vi "EditorDaemon openFile.vi"(8 "error in (no error)":errorcluster, 9 "dataName":string(combo) caption="Data Name", 10 "filePath":path caption="File Path") -> (0 "error out":errorcluster, 1 "dataName out":string caption="Data Name", 2 "currFilePath":path, 3 "signal out":waveform(sgl), 4 "update":bool)   [LabVIEW 2018]
uses:
  PC/PublicSubVI/Class/FileManager/FM/ctl/_PC_Pub_FM fileReadFuncEnum.ctl
  PC/PublicSubVI/Class/FileManager/TDMSAdv.lvclass
panel:
  out "remark":string caption="Data Remark"
  in  "cancelBtn":bool
  in  "loadBtn":bool
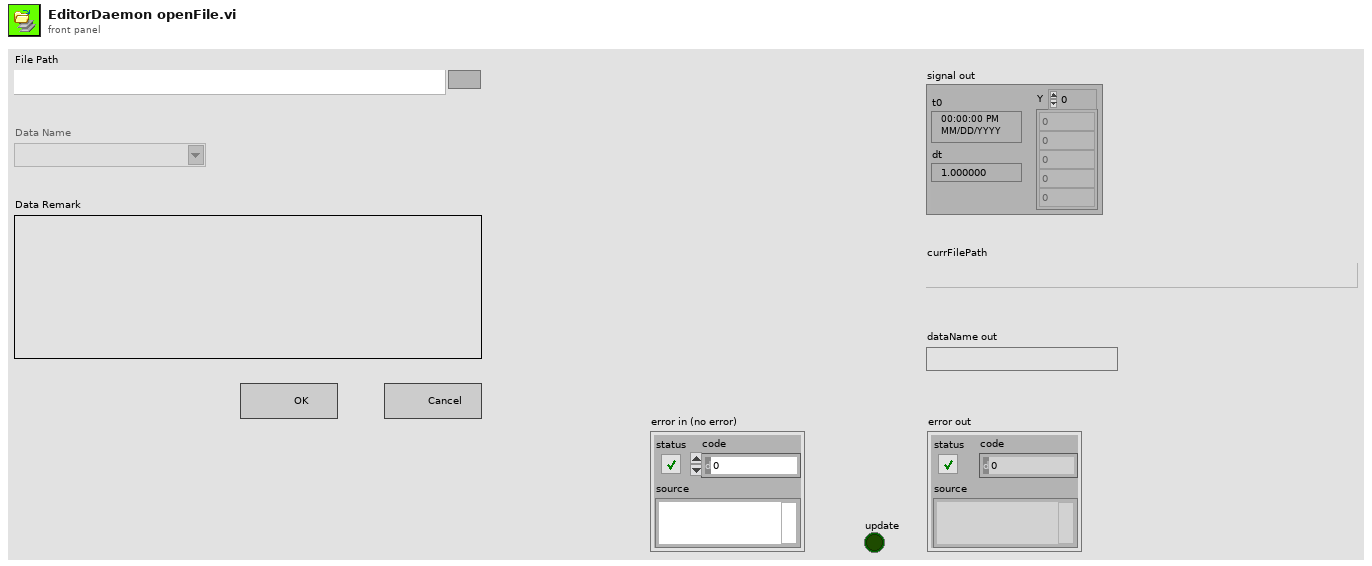
[diagram p1: front panel]
types:
  T1 = enum8{"Enabled", "Disabled", "Disabled and Grayed Out"}
  T2 = enum16{"open", "open or create", "create or replace", "create", "open (read-only)"}
  T3 = typedef "_PC_Pub_FM fileReadFuncEnum.ctl" = enum16{"getAllInfo", "getChromatogram", "getDataItems", "getTimeStamp", "getIdxData", "getIonization", "getRemark", "getAttrFormat"}
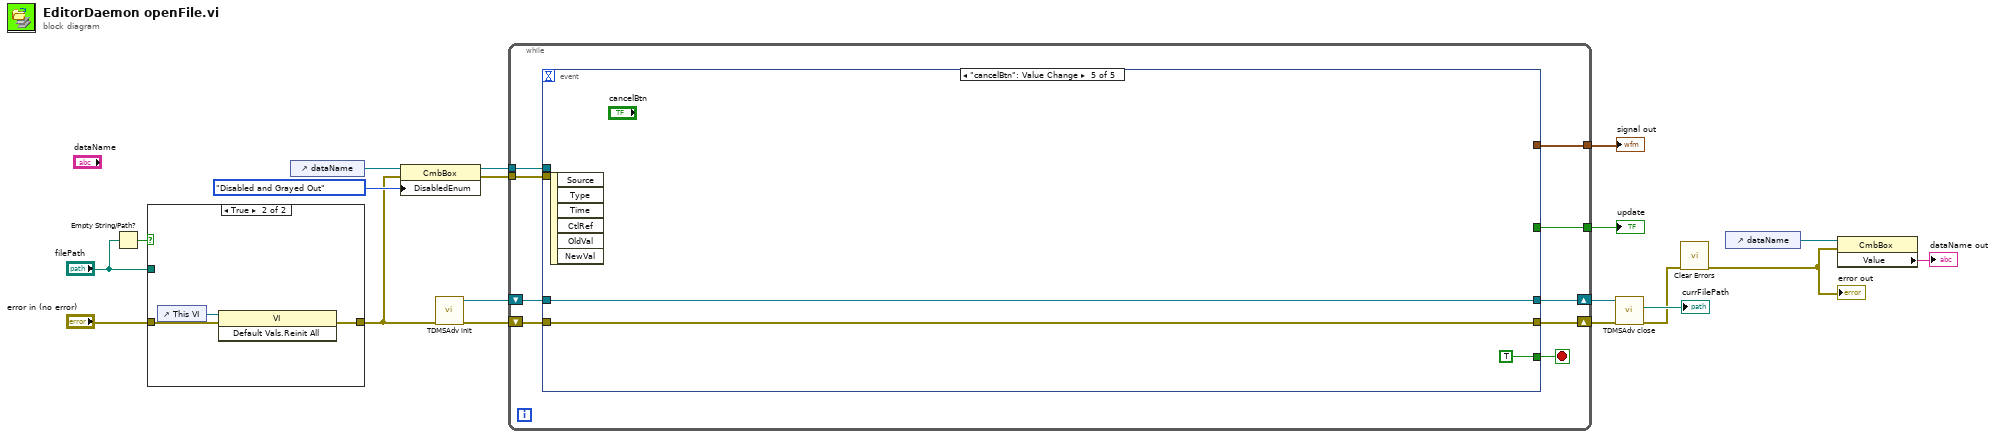
[diagram p0: block diagram]
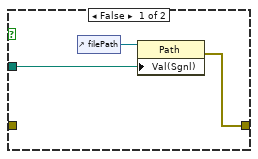
[diagram p2: hidden frame]
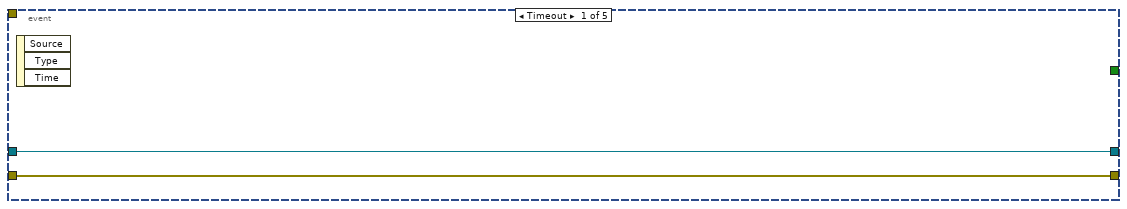
[diagram p3: hidden frame]
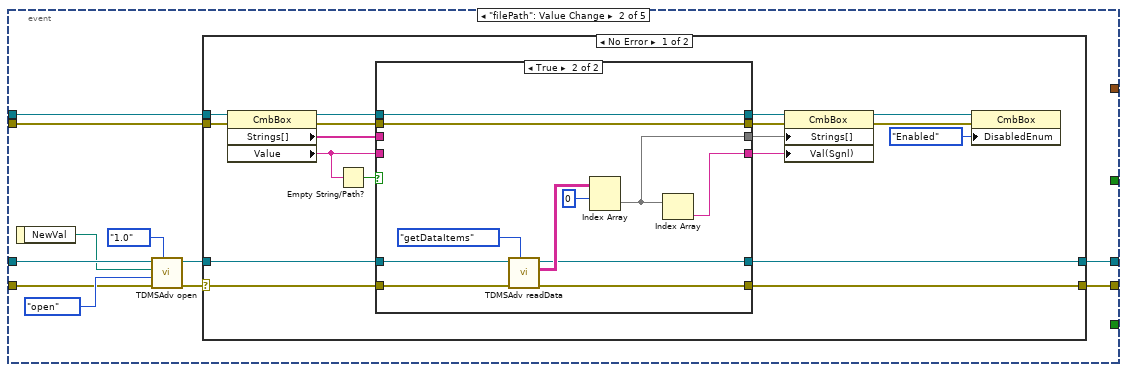
[diagram p4: hidden frame]
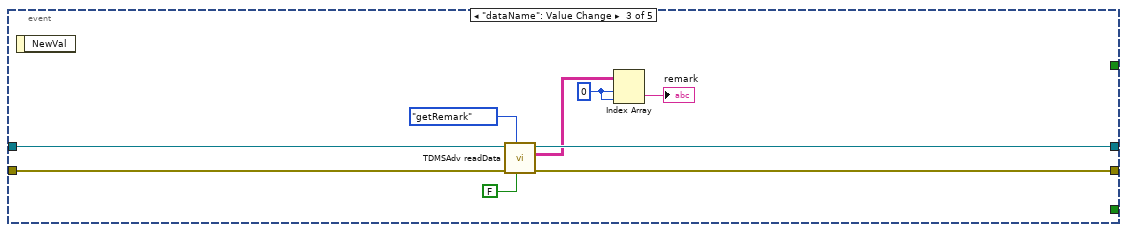
[diagram p7: hidden frame]
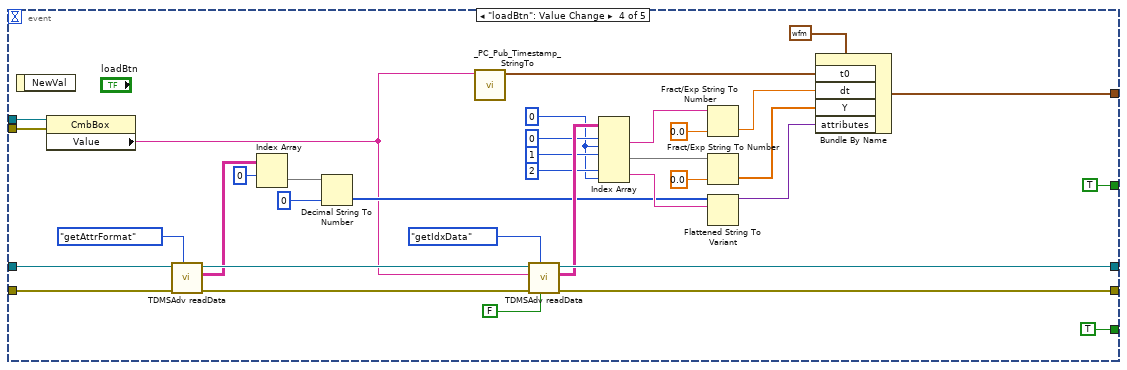
[diagram p8: hidden frame]
diagram:
  n1 = Empty String/Path?(string/path="filePath") -> (empty?=w10:bool)
  n2 = case shown="True" w10 {
    tunnel: "filePath" -> [w22 _]
    tunnel: [w20 w23] -> w6
    tunnel: "error in (no error)" -> [_ w24]
    frame False {
      n3 = control-ref of="filePath"() -> (w21:refnum<vi>)
      n4 = property class="Path"(reference=w21, "Val(Sgnl)"=w22) -> (error out=w20:errorcluster)  [unwired: 1 in, 1 out]
    }
    frame True {
      n5 = control-ref of="This VI"() -> (w25:refnum<vi>)
      n6 = invoke class="VI" method="Default Vals.Reinit All"(reference=w25, error in=w24) -> (error out=w23:errorcluster)  [unwired: 1 in, 2 out]
    }
  }
  n7 = control-ref of="dataName"() -> (w13:refnum<vi>)
  n8 = property class="CmbBox"(reference=w13, error in=w6, "DisabledEnum"=T1."Disabled and Grayed Out" ("Disabled")) -> (reference out=w12:refnum<vi>, error out=w11:errorcluster)
  n9 = call "TDMSAdv init.vi"("error in (no error)"=w6) -> ("error out"=w18:errorcluster, "TDMSAdv out"=w19:refnum<class "TDMSAdv.lvclass">)  [unwired: 9 in]
  n10 = while {
    tunnel: w11 -> [w32]
    tunnel: w12 -> [w33]
    shift-right: [w29] -> w17
    shift-left: w19 -> [w30]
    shift-right: [w28] -> w3
    shift-left: w18 -> [w31]
    tunnel: [w27] -> w16
    tunnel: [w26] -> w9
    stop <- w34 stop-if-true
    n11 = event shown="[4] \"cancelBtn\": Value Change" {
      selector: _ -> [_ _ _ _ _]
      dyn-events: _ -> [_ _ _ _ _]
      timeout: _ -> [_ _ _ _ _]
      tunnel: [_ _ _ TRUE TRUE] -> w34
      tunnel: w33 -> [_ w47 _ w126 _]
      tunnel: w32 -> [_ w46 _ w125 _]
      tunnel: w31 -> [w35 w42 w90 w121 w128]
      tunnel: w30 -> [w36 w43 w91 w122 w129]
      tunnel: [w36 w40 w89 w123 w129] -> w29
      tunnel: [w35 w39 w88 w124 w128] -> w28
      tunnel: [_ _ _ w94 _] -> w27
      tunnel: [_ _ _ TRUE _] -> w26
      event Timeout {
        n12 = event-data() -> ()  [unwired: 1 in, 3 out]
      }
      event "filePath": Value Change {
        n13 = event-data() -> ("NewVal"=w37:path)  [unwired: 1 in]
        n14 = call "TDMSAdv open.vi"("file format version"=enum16{"1.0", "2.0", "Adv"}."1.0", "error in (no error)"=w42, "operation (0:open)"=T2."open", "openPath"=w37, "TDMSAdv in"=w43) -> ("error out"=w38:errorcluster, "TDMSAdv out"=w41:refnum<class "TDMSAdv.lvclass">)  [unwired: 5 in]
        n15 = case shown="No Error" w38 {
          selector: w38 -> [w57 _]
          tunnel: w47 -> [w56 _]
          tunnel: w46 -> [w55 _]
          tunnel: w41 -> [w61 w83]
          tunnel: [w59 w83] -> w40
          tunnel: [w58 _] -> w39
          frame No Error {
            n16 = property class="CmbBox"(reference=w56, error in=w55) -> (reference out=w52:refnum<vi>, error out=w50:errorcluster, "Strings[]"=w49:string[], "Value"=w48:string)
            n17 = Empty String/Path?(string/path=w48) -> (empty?=w54:bool)
            n18 = case shown="True" w54 {
              tunnel: [w68 w82] -> w62
              tunnel: w61 -> [w67 w81]
              tunnel: [w71 w79] -> w60
              tunnel: [w67 w78] -> w59
              tunnel: [w66 w77] -> w58
              tunnel: w57 -> [w66 w74]
              tunnel: w48 -> [w68 _]
              tunnel: [w70 w73] -> w53
              tunnel: w52 -> [w70 w73]
              tunnel: [w69 w72] -> w51
              tunnel: w50 -> [w69 w72]
              tunnel: w49 -> [w71 _]
              frame False {
              }
              frame True {
                n19 = call "TDMSAdv readData.vi"("readEvent"=_PC_Pub_FM_fileReadFuncEnum."getDataItems", "error in (no error)"=w74, "TDMSAdv in"=w81) -> ("error out"=w77:errorcluster, "outputArr"=w80:string[][], "TDMSAdv out"=w78:refnum<class "TDMSAdv.lvclass">)  [unwired: 5 in, 1 out]
                n20 = Index Array(array=w80, index (row)=0 ("disabled index (col)")) -> (element=w79:string[])  [unwired: 1 in]
                n21 = Index Array(array=w79) -> (element=w82:string)  [unwired: 1 in]
              }
            }
            n22 = property class="CmbBox"(reference=w53, error in=w51, "Strings[]"=w60, "Val(Sgnl)"=w62) -> (reference out=w65:refnum<vi>, error out=w64:errorcluster)
            n23 = property class="CmbBox"(reference=w65, error in=w64, "DisabledEnum"=T1."Enabled" ("Disabled")) -> ()  [unwired: 2 out]
          }
          frame Error {
          }
        }
      }
      event "dataName": Value Change {
        w86 = 0 ("index (row)")
        n24 = event-data() -> ()  [unwired: 1 in, 1 out]
        n25 = call "TDMSAdv readData.vi"("stringSplit? (T)"=FALSE, "readEvent"=_PC_Pub_FM_fileReadFuncEnum."getRemark", "error in (no error)"=w90, "TDMSAdv in"=w91) -> ("error out"=w88:errorcluster, "outputArr"=w87:string[][], "TDMSAdv out"=w89:refnum<class "TDMSAdv.lvclass">)  [unwired: 4 in, 1 out]
        n26 = Index Array(array=w87, index (row)=w86, index (col)=w86) -> (element=→"remark":string)
      }
      event "loadBtn": Value Change {
        w110 = 0 ("disabled index (col)")
        n27 = event-data() -> ()  [unwired: 1 in, 1 out]
        n28 = property class="CmbBox"(reference=w126, error in=w125) -> ("Value"=w103:string)  [unwired: 2 out]
        n29 = call "TDMSAdv readData.vi"("readEvent"=_PC_Pub_FM_fileReadFuncEnum."getAttrFormat", "error in (no error)"=w121, "TDMSAdv in"=w122) -> ("error out"=w120:errorcluster, "outputArr"=w115:string[][], "TDMSAdv out"=w119:refnum<class "TDMSAdv.lvclass">)  [unwired: 5 in, 1 out]
        n30 = Index Array(array=w115, index (row)=0) -> (element=w116:string[])  [unwired: 1 in]
        n31 = Decimal String To Number(string=w116, default (0L)=i16 0 ("default (0 I32)")) -> (number=w106:i16[])  [unwired: 1 in, 1 out]
        n32 = call "_PC_Pub_Timestamp_StringTo.vi"("Timestring"=w103) -> ("Timestamp"=w101:timestamp)  [unwired: 9 in, 1 out]
        n33 = call "TDMSAdv readData.vi"("stringSplit? (T)"=FALSE, "readEvent"=_PC_Pub_FM_fileReadFuncEnum."getIdxData", "error in (no error)"=w120, "timeStamp"=w103, "TDMSAdv in"=w119) -> ("error out"=w124:errorcluster, "outputArr"=w114:string[][], "TDMSAdv out"=w123:refnum<class "TDMSAdv.lvclass">)  [unwired: 3 in, 1 out]
        n34 = Index Array(array=w114, index (row) #1=0 ("index (row)"), index (col) #1=w110, index (row) #2=1 ("index (row)"), index (row) #3=2 ("index (row)"), index (col) #3=w110) -> (element #1=w108:string, element #2=w109:string[], element #3=w107:string)  [unwired: 1 in]
        n35 = Fract/Exp String To Number(string=w108, default (0 dbl)=0.0 ("default (0 DBL)")) -> (number=w100:dbl)  [unwired: 2 in, 1 out]
        n36 = Fract/Exp String To Number(string=w109, default (0 dbl)=sgl 0.0 ("default (0 DBL)")) -> (number=w99:sgl[])  [unwired: 2 in, 1 out]
        n37 = Flattened String To Variant(6:w107, 7:w106) -> (3:w98:variant)  [unwired: 1 in, 1 out]
        n38 = Bundle By Name(cluster=waveform(sgl) {"t0"=timestamp(0 s since 1904-01-01), "dt"=1.0, "Y"=[]} ("signal in"), "t0"=w101, "dt"=w100, "Y"=w99, "attributes"=w98) -> (w94:waveform(sgl))
      }
      event "cancelBtn": Value Change {
        n39 = event-data() -> ()  [unwired: 1 in, 6 out]
      }
    }
  }
  "signal out" <- w16
  "update" <- w9
  n40 = call "TDMSAdv close.vi"("error in (no error)"=w3, "TDMSAdv in"=w17) -> ("error out"=w2:errorcluster, "filePath"=→"currFilePath":path)  [unwired: 7 in, 1 out]
  n41 = call <vilib>:"Clear Errors.vi"("error in (no error)"=w2) -> ("error out"=w1:errorcluster)  [unwired: 5 in, 1 out]
  "error out" <- w1
  n42 = control-ref of="dataName"() -> (w5:refnum<vi>)
  n43 = property class="CmbBox"(reference=w5, error in=w1) -> ("Value"=→"dataName out":string)  [unwired: 2 out]
